vi "EFMC-6.vi"(11 "数组":u8[](array[numeric])) -> (0 "通讯状态":bool=TRUE, 1 "字符串":string, 2 "系统单次上电工作时间":dbl, 3 "北京时间":timestamp)   [LabVIEW 2012]
uses:
  index-i8.vi
  index-i32.vi
  XX-DBL.vi
  index-dbl.vi
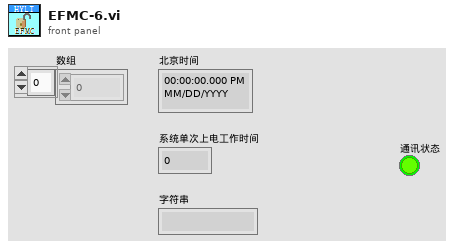
[diagram p1: front panel]
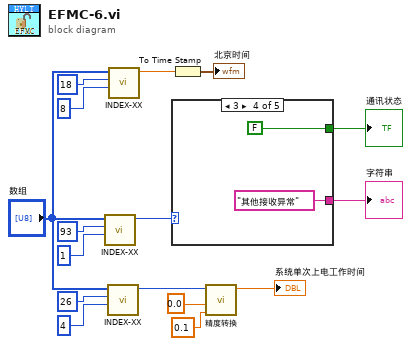
[diagram p0: block diagram]
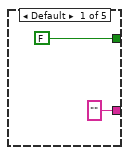
[diagram p2: hidden frame]
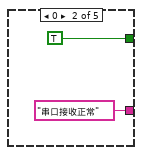
[diagram p3: hidden frame]
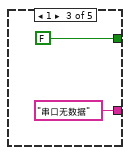
[diagram p4: hidden frame]
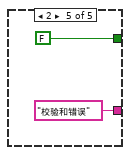
[diagram p5: hidden frame]
diagram:
  n1 = call-poly "INDEX-XX.vi"("长度"=1, "索引"=93, "数组"="数组") -> ("数值输出"=w15:i8)  [unwired: 8 in]
  n2 = call-poly "INDEX-XX.vi"("长度"=4, "索引"=26, "数组"="数组") -> ("数值输出"=w8:i32)  [unwired: 8 in]
  n3 = call-poly "INDEX-XX.vi"("长度"=8, "索引"=18, "数组"="数组") -> ("数值输出"=w2:dbl)  [unwired: 8 in]
  n4 = case shown="3" w15 {
    tunnel: ["" "串口接收正常" "串口无数据" "其他接收异常" "校验和错误"] -> w16
    tunnel: [FALSE TRUE FALSE FALSE FALSE] -> w1
    frame Default {
    }
    frame 0 {
    }
    frame 1 {
    }
    frame 3 {
    }
    frame 2 {
    }
  }
  "字符串" <- w16
  "通讯状态" <- w1
  n5 = To Time Stamp(1:w2) -> (0:→"北京时间":timestamp)
  n6 = call-poly "精度转换.vi"("单位"=0.1, "下限"=0.0, "数值输入"=w8) -> ("输出"=→"系统单次上电工作时间":dbl)  [unwired: 8 in]
